vi "niRFSTS Digital Configure digital and disconnected.vi"(0 "Semiconductor Module Context":T1, 5 "Pin Names":string[](array[string]), 11 "error in (no error)":errorcluster) -> (15 "error out":errorcluster)   [LabVIEW 2014]
uses:
  <vilib>/NI_TestStand_SemiconductorModule/NI_TestStand_Semiconductor_Module.lvlibp/PinMap/General/SemiconductorModuleContext.ctl
  <instrlib>/niDigital/niDigital.llb/niDigital Selected Function.ctl
  <instrlib>/niDigital/niDigital.llb/niDigital Write Static Pin State.ctl
  <vilib>/NI_TestStand_SemiconductorModule/NI_TestStand_Semiconductor_Module.lvlibp/PinMap/Digital Pattern/PinsToNIDigitalPatternSessions.vi
  <vilib>/NI_TestStand_SemiconductorModule/NI_TestStand_Semiconductor_Module.lvlibp
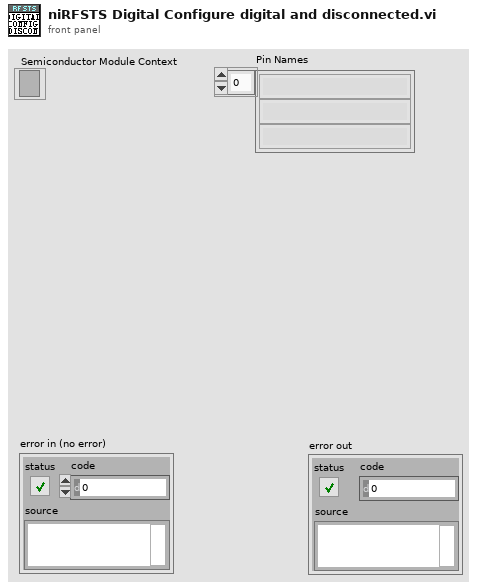
[diagram p1: front panel]
types:
  T1 = typedef "NI_TestStand_Semiconductor_Module.lvlibp/SemiconductorModuleContext.ctl" = refnum<k7>
  T2 = typedef "niDigital Selected Function.ctl" = i32
  T3 = typedef "niDigital Write Static Pin State.ctl" = u8
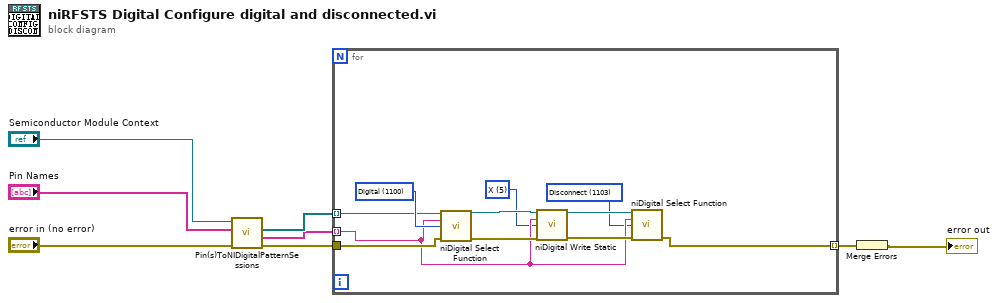
[diagram p0: block diagram]
diagram:
  n1 = call-poly <vilib>:"Pin(s)ToNIDigitalPatternSessions.vi"("error in (no error)"="error in (no error)", "Pins"="Pin Names", "Semiconductor Module Context"="Semiconductor Module Context") -> ("error out"=w3:errorcluster, "Channel Lists"=w6:string[], "Instrument Sessions"=w7:refnum<k15>[])  [unwired: 3 in, 3 out]
  n2 = for {
    tunnel: w7 -> [w18] mode=indexing
    tunnel: w6 -> [w13] mode=indexing
    tunnel: w3 -> [w17]
    tunnel: [w9] -> w2 mode=indexing
    w12 = T2 1103 items=["Digital"=1100, "PPMU"=1101, "Off"=1102, "Disconnect"=1103] ("function")
    w10 = T3 5 items=["0"=0, "1"=1, "X"=5] ("state")
    w19 = T2 1100 items=["Digital"=1100, "PPMU"=1101, "Off"=1102, "Disconnect"=1103] ("function")
    n3 = call <instrlib>:"niDigital Select Function.vi"("instrument handle"=w18, "channel list"=w13, "function"=w19, "error in"=w17) -> ("instrument handle out"=w11:refnum<k15>, "error out"=w16:errorcluster)  [unwired: 10 in]
    n4 = call <instrlib>:"niDigital Write Static.vi"("instrument handle"=w11, "channel list"=w13, "state"=w10, "error in"=w16) -> ("instrument handle out"=w14:refnum<k15>, "error out"=w15:errorcluster)  [unwired: 10 in]
    n5 = call <instrlib>:"niDigital Select Function.vi"("instrument handle"=w14, "channel list"=w13, "function"=w12, "error in"=w15) -> ("error out"=w9:errorcluster)  [unwired: 10 in, 1 out]
  }
  n6 = Merge Errors(w2) -> (→"error out":errorcluster)
